vi "OrthogonalMatchingPursuitCV.vi"(8 "error in":errorcluster) -> (0 "error out":errorcluster, 3 "out":refnum<class "OrthogonalMatchingPursuitCV.lvclass">)   [LabVIEW 2020]
doc: "Cross-validated Orthogonal Matching Pursuit model (OMP).\n\n See glossary entry for :term:`cross-validation estimator`.\n\n Read more in the :ref:`User Guide <omp>`.\n\n Parameters\n ----------\n copy : bool, default=True\n Whether the design matrix X must be copied by the algorithm. A false\n value is only helpful if X is already Fortran-ordered, otherwise a\n copy is made anyway.\n\n fit_intercept : bool, default=True\n whether to calculate the intercept for this model. If set\n to false, no intercept will be used in calculations\n (i.e. data is expected to be centered).\n\n normalize : bool, default=True\n This parameter is ignored when ``fit_intercept`` is set to False.\n If True, the regressors X will be normalized before regression by\n subtracting the mean and dividing by the l2-norm.\n If you wish to standardize, please use\n :class:`~sklearn.preprocessing.StandardScaler` before calling ``fit``\n on an estimator with ``normalize=False``.\n\n max_iter : int, default=None\n Maximum numbers of iterations to perform, therefore maximum features\n to include. 10% of ``n_features`` but at least 5 if available.\n\n cv : int, cross-validation generator or iterable, default=None\n Determines the cross-validation splitting strategy.\n Possible inputs for cv are:\n\n - None, to use the default 5-fold cross-validation,\n - integer, to specify the number of folds.\n - :term:`CV splitter`,\n - An iterable yielding (train, test) splits as arrays of indices.\n\n For integer/None inputs, :class:`KFold` is used.\n\n Refer :ref:`User Guide <cross_validation>` for the various\n cross-validation strategies that can be used here.\n\n .. versionchanged:: 0.22\n ``cv`` default value if None changed from 3-fold to 5-fold.\n\n n_jobs : int, default=None\n Number of CPUs to use during the cross validation.\n ``None`` means 1 unless in a :obj:`joblib.parallel_backend` context.\n ``-1`` means using all processors. See :term:`Glossary <n_jobs>`\n for more details.\n\n verbose : bool or int, default=False\n Sets the verbosity amount.\n\n Attributes\n ----------\n intercept_ : float or ndarray of shape (n_targets,)\n Independent term in decision function.\n\n coef_ : ndarray of shape (n_features,) or (n_targets, n_features)\n Parameter vector (w in the problem formulation).\n\n n_nonzero_coefs_ : int\n Estimated number of non-zero coefficients giving the best mean squared\n error over the cross-validation folds.\n\n n_iter_ : int or array-like\n Number of active features across every target for the model refit with\n the best hyperparameters got by cross-validating across all folds.\n\n \nAvailable methods:\nGet Attributes\nGet Params\nSet Params"
uses:
  OrthogonalMatchingPursuitCV.lvclass
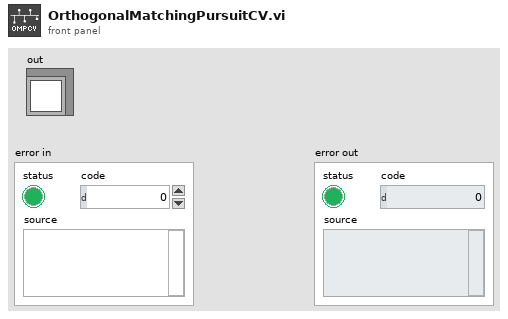
[diagram p1: front panel]
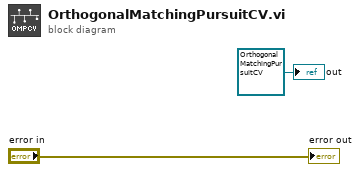
[diagram p0: block diagram]
diagram:
  "out" <- refnum<class "OrthogonalMatchingPursuitCV.lvclass"> refnum ("model")
  "error out" <- "error in"
